vi "Read trigger modifier (None).vi"(8 "error in (no error)":errorcluster, 11 "Configure Trigger Modifier [TM] Msg in":refnum<class "Configure Trigger Modifier [TM] Msg.lvclass">) -> (0 "error out":errorcluster, 2 "trigger modifier (None)":i32(ring)=1 items=["None"=1, "Auto"=2, "Auto Level"=3], 3 "Configure Trigger Modifier [TM] Msg out":refnum<class "Configure Trigger Modifier [TM] Msg.lvclass">)   [LabVIEW 2015, in "CS++Scope.lvlib" / "Configure Trigger Modifier [TM] Msg.lvclass"]
uses:
  Configure Trigger Modifier [TM] Msg.lvclass
  Configure Trigger Modifier [TM] Msg.lvclass/Configure Trigger Modifier [TM] Msg.ctl
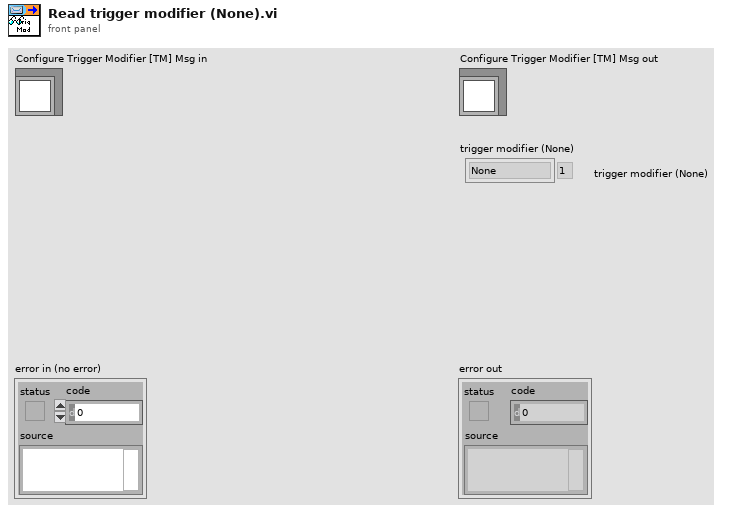
[diagram p1: front panel]
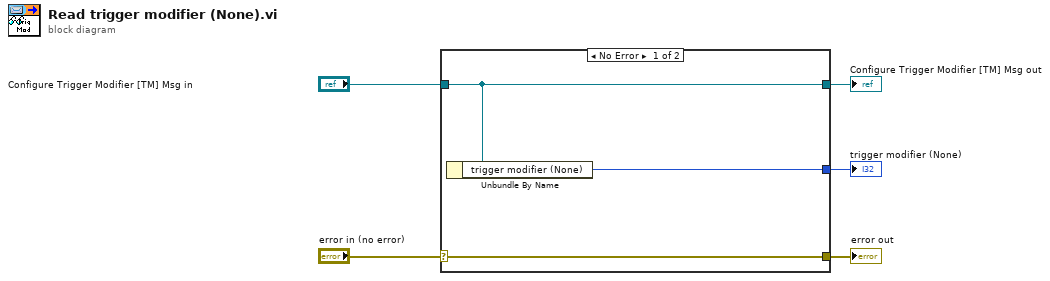
[diagram p0: block diagram]
diagram:
  n1 = case shown="No Error" "error in (no error)" {
    selector: "error in (no error)" -> [w8 w9]
    tunnel: [w8 w9] -> w4
    tunnel: [w7 w10] -> w2
    tunnel: "Configure Trigger Modifier [TM] Msg in" -> [w7 w10]
    tunnel: [w6 _] -> w1
    frame No Error {
      n2 = Unbundle By Name(w7) -> ("trigger modifier (None)"=w6:i32)
    }
    frame Error {
    }
  }
  "error out" <- w4
  "Configure Trigger Modifier [TM] Msg out" <- w2
  "trigger modifier (None)" <- w1
